vi "Read Bounds Area Width.vi"(8 "error in (no error)":errorcluster, 11 "GObject.lvclass in":refnum<class "GObject.lvclass">) -> (0 "error out":errorcluster, 2 "Area Width":u32, 3 "GObject.lvclass out":refnum<class "GObject.lvclass">)   [LabVIEW 2015, in "GObject.lvclass"]
uses:
  GObject.lvclass
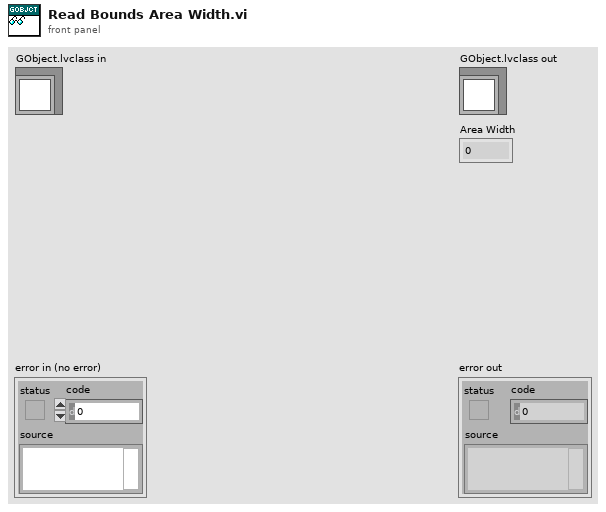
[diagram p1: front panel]
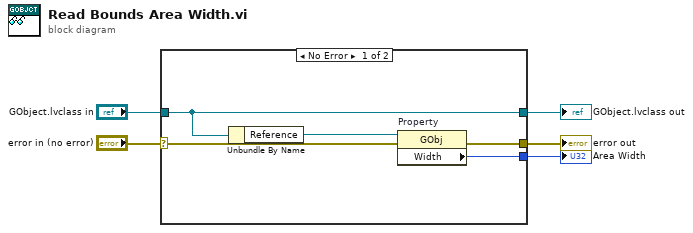
[diagram p0: block diagram]
diagram:
  n1 = case shown="No Error" "error in (no error)" {
    selector: "error in (no error)" -> [w6 w12]
    tunnel: [w9 w12] -> w4
    tunnel: [w8 w11] -> w2
    tunnel: "GObject.lvclass in" -> [w8 w11]
    tunnel: [w10 _] -> w1
    frame No Error {
      n2 = Unbundle By Name(w8) -> ("Reference"=w7:refnum<vi>)
      n3 = property on="Property" class="GObj"(reference=w7, error in=w6) -> (error out=w9:errorcluster, "Width"=w10:u32)  [unwired: 1 out]
    }
    frame Error {
    }
  }
  "error out" <- w4
  "GObject.lvclass out" <- w2
  "Area Width" <- w1
